vi "模拟输入_热电偶_软件按需单点.vi"() -> ()   [LabVIEW 2013]
doc: "该范例演示了使用DAQmx设备连续采集热电偶测量的方法。\n\n关于连接信号至DAQ设备的方法，请查看设备文档。"
uses:
  <vilib>/Utility/error.llb/DialogType.ctl
  <userlib>/ArtDAQ/_SubVI/ArtDAQ_CreateAIThrmcplChan.vi
  <userlib>/ArtDAQ/_SubVI/ArtDAQ_Read Analog DBL NChan 1Samp.vi
panel:
  in  "归零类型":i32(ring)=2 items=["禁用", "单次归零", "每次归零"]
  in  "CJC通道":string
  in  "CJC值":dbl=25.0 format="%0.2f"
  in  "CJC源":i32(ring)=10116 items=["内置"=10200, "常量值"=10116, "通道"=10113]
  in  "热电偶类型":i32(ring)=10072 items=["J"=10072, "k"=10073, "N"=10077, "R"=10082, "S"=10085, "T"=10086, "B"=10047, "E"=10055]
  in  "单位":i32(ring)=10143 items=["Deg C"=10143, "Deg F"=10144, "Kelvins"=10325, "Deg R"=10145, "来自自定义换算"=10065]
  in  "循环时间(ms)":u32=100
  in  "停止":bool
  in  "最高温度":dbl=100.0
  in  "最低温度":dbl
  in  "物理通道":string="Dev1/ai0"
  out "波形图表":dbl[][](graph)
  # "采集数据"
  # "通道设置"
  # "定时设置"
  # "自动归零设置"
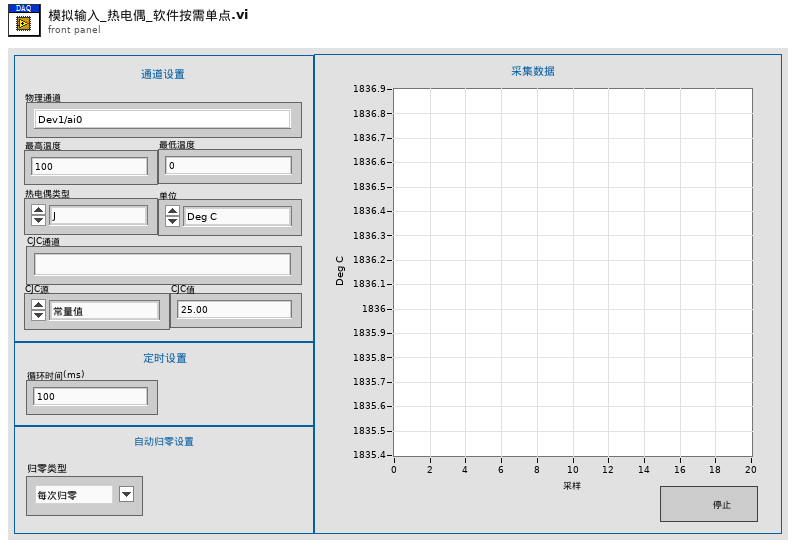
[diagram p1: front panel]
types:
  T1 = typedef "DialogType.ctl" = u16
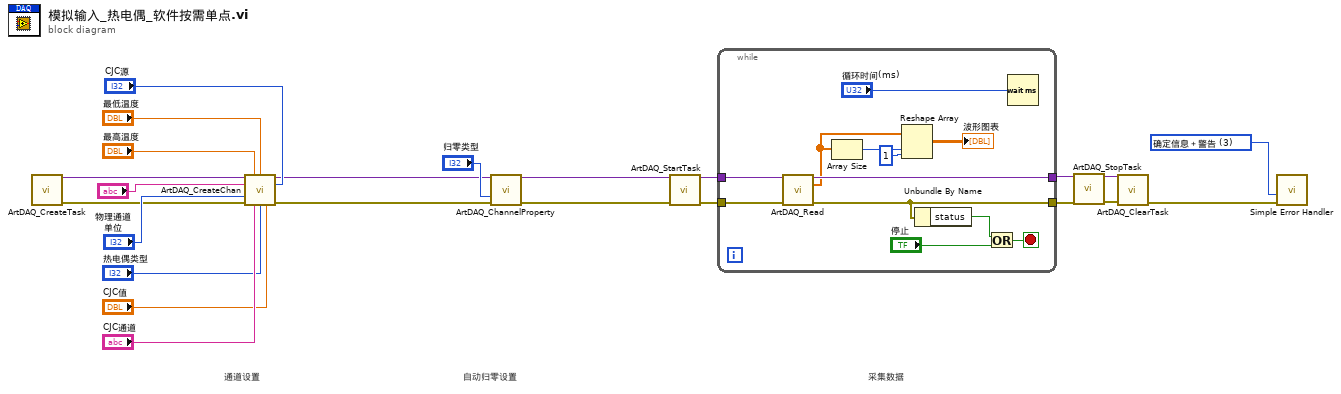
[diagram p0: block diagram]
diagram:
  w16 = T1 3 items=["无对话框", "确定信息", "继续或停止信息", "确定信息＋警告", "继续/停止＋警告"] ("对话框类型（确定信息：1）")
  # "自动归零设置"
  # "采集数据"
  # "通道设置"
  n1 = call <userlib>:"ArtDAQ_CreateTask.vi"() -> ("任务句柄"=w2:variant, "错误输出"=w1:errorcluster)  [unwired: 14 in]
  n2 = call-poly <userlib>:"ArtDAQ_CreateChan.vi"("任务句柄"=w2, "最大值"="最高温度", "最小值"="最低温度", "物理通道"="物理通道", "CJC源"="CJC源", "单位"="单位", "错误输入"=w1, "CJC通道"="CJC通道", "热电偶类型"="热电偶类型", "CJC值"="CJC值") -> ("任务句柄"=w6:variant, "错误输出"=w5:errorcluster)  [unwired: 4 in]
  n3 = call-poly <userlib>:"ArtDAQ_ChannelProperty.vi"("任务句柄"=w6, "归零类型"="归零类型", "错误输入"=w5) -> ("任务句柄"=w4:variant, "错误输出"=w3:errorcluster)  [unwired: 11 in]
  n4 = call <userlib>:"ArtDAQ_StartTask.vi"("任务句柄"=w4, "错误输入"=w3) -> ("任务句柄"=w23:variant, "错误输出"=w22:errorcluster)  [unwired: 12 in]
  n5 = while {
    tunnel: w23 -> [w35]
    tunnel: w22 -> [w34]
    tunnel: [w31] -> w17
    tunnel: [w32] -> w18
    stop <- w33 stop-if-true
    n6 = call-poly <userlib>:"ArtDAQ_Read.vi"("任务句柄"=w35, "错误输入"=w34) -> ("任务句柄"=w32:variant, "数据"=w27:dbl[], "错误输出"=w31:errorcluster)  [unwired: 11 in]
    n7 = Array Size(array=w27) -> (size(s)=w26:i32)
    n8 = Reshape Array(w27, w26, 1 ("维数大小")) -> (→"波形图表":dbl[][])
    n9 = Unbundle By Name(w31) -> ("status"=w30:bool)
    n10 = Or(x=w30, y="停止") -> (x .or. y?=w33:bool)
    n11 = Wait (ms)(milliseconds to wait="循环时间(ms)") -> ()  [unwired: 1 out]
  }
  n12 = call <userlib>:"ArtDAQ_StopTask.vi"("任务句柄"=w18, "错误输入"=w17) -> ("任务句柄"=w20:variant, "错误输出"=w19:errorcluster)  [unwired: 12 in]
  n13 = call <userlib>:"ArtDAQ_ClearTask.vi"("任务句柄"=w20, "错误输入"=w19) -> ("错误输出"=w21:errorcluster)  [unwired: 13 in]
  n14 = call <vilib>:"Simple Error Handler.vi"("type of dialog (OK msg:1)"=w16, "error in (no error)"=w21) -> ()  [unwired: 3 in, 5 out]
